vi "题目7.vi"() -> ()   [LabVIEW 2017]
uses:
  <vilib>/Utility/file.llb/Read Delimited Spreadsheet (DBL).vi
  <vilib>/Analysis/NI_AALBase.lvlib
panel:
  out "波形图表":dbl(graph)
  out "all rows":dbl[][](array[numeric]) caption="所有行"
  in  "cycles":dbl=1.0 caption="周期" format="%0.2f"
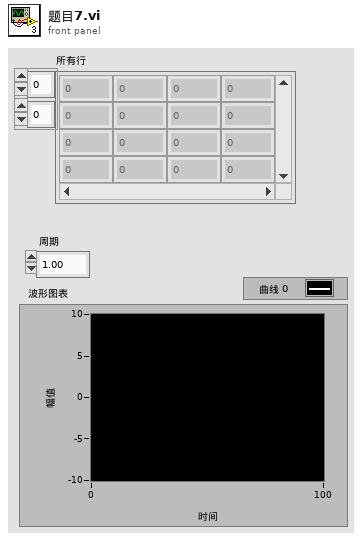
[diagram p1: front panel]
types:
  T1 = enum16{"open", "replace", "create", "open or create", "replace or create", "replace or create with confirmation"}
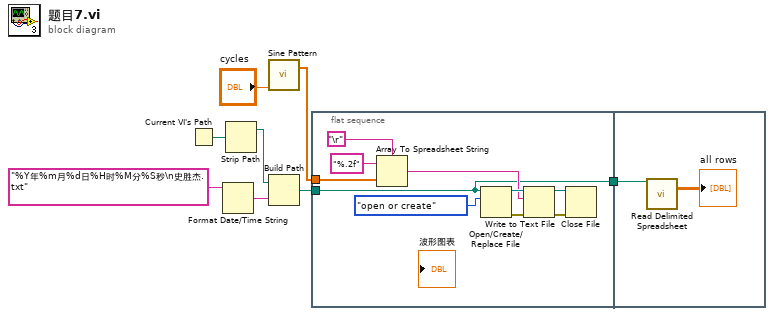
[diagram p0: block diagram]
diagram:
  n1 = Current VI's Path() -> (path=w8:path)
  n2 = Format Date/Time String(time format string (%c)="%Y年%m月%d日%H时%M分%S秒\n史胜杰.txt") -> (date/time string=w7:string)  [unwired: 2 in]
  n3 = Strip Path(path=w8) -> (stripped path=w6:path)  [unwired: 1 out]
  n4 = call <vilib>:"Sine Pattern.vi"("cycles"="cycles") -> ("Sinusoidal Pattern"=w2:dbl[])  [unwired: 3 in, 1 out]
  n5 = Build Path(base path=w6, name or relative path=w7) -> (appended path=w3:path)
  n6 = flat-sequence {
    tunnel: w3 -> [w9]
    tunnel: w2 -> [w13]
    tunnel: [w9] -> w1
    tunnel: w1 -> [w20]
    frame #0 {
      n7 = Array To Spreadsheet String(delimiter (Tab)="\r", array=w13, 3:"%.2f" ("格式字符串")) -> (spreadsheet string=w10:string)
      n8 = Open/Create/Replace File(file path (use dialog)=w9, operation (0:open)=T1."open or create" ("操作(0:open)")) -> (refnum out=w15:refnum<file>, error out=w18:errorcluster)  [unwired: 4 in, 1 out]
      n9 = Write to Text File(file (use dialog)=w15, text=w10, error in=w18) -> (refnum out=w16:refnum<file>, error out=w17:errorcluster)  [unwired: 1 in, 1 out]
      n10 = Close File(refnum=w16, error in=w17) -> ()  [unwired: 2 out]
    }
    frame #1 {
      n11 = call-poly <vilib>:"Read Delimited Spreadsheet.vi"("file path (dialog if empty)"=w20) -> ("all rows"=→"all rows":dbl[][])  [unwired: 9 in, 5 out]
    }
  }
